vi "Data_1D_with_IgorX.vi"(6 "Data From Igor":bool, 8 "error in (no error)":errorcluster, 9 "Wave Name":string, 10 "Wave Prefix":string, 11 "1D Data IN":dbl[](array[numeric])) -> (0 "error out":errorcluster, 2 "Wave Prefix Through":string, 3 "1D Data OUT":dbl[](array[numeric]))   [LabVIEW 2014]
panel:
  in  "Igor Application IN":refnum<k7>
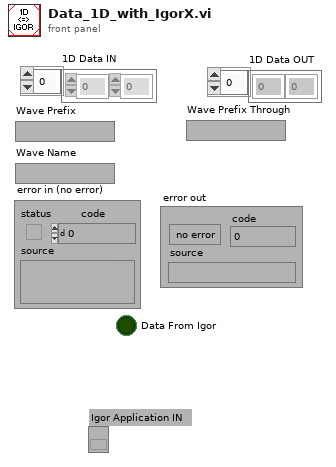
[diagram p1: front panel]
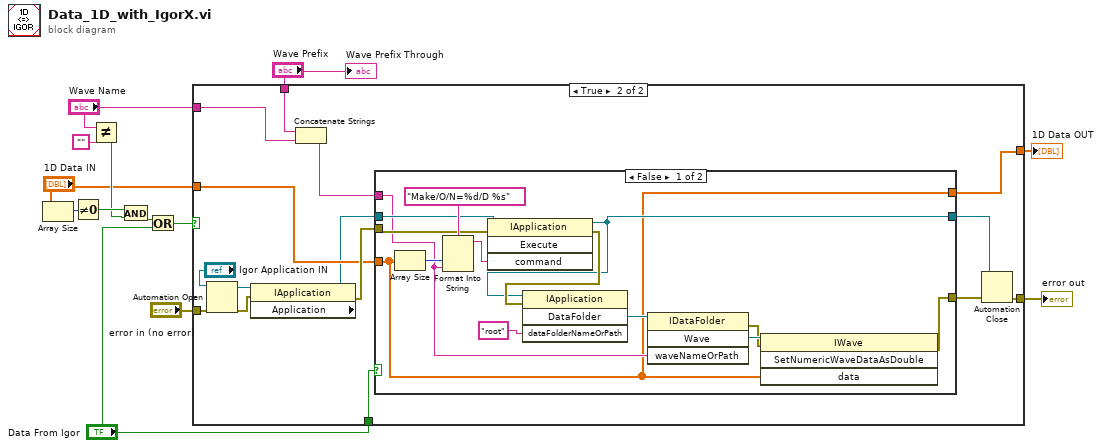
[diagram p0: block diagram]
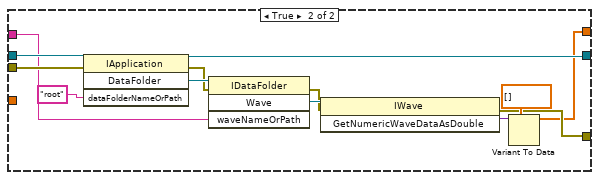
[diagram p3: hidden frame]
diagram:
  n1 = Array Size(array="1D Data IN") -> (size(s)=w13:i32)
  n2 = Not Equal To 0?(x=w13) -> (x != 0?=w12:bool)
  n3 = Not Equal?(x="Wave Name", y="") -> (x != y?=w9:bool)
  n4 = And(x=w12, y=w9) -> (x .and. y?=w3:bool)
  n5 = Or(x=w3, y="Data From Igor") -> (x .or. y?=w2:bool)
  n6 = case shown="True" w2 {
    tunnel: "1D Data IN" -> [w14 w17]
    tunnel: "Wave Name" -> [_ w29]
    tunnel: "Wave Prefix" -> [_ w30]
    tunnel: "error in (no error)" -> [w15 w24]
    tunnel: [w15 w22] -> w7
    tunnel: "Data From Igor" -> [_ w28]
    tunnel: [w14 w18] -> w4
    frame False {
    }
    frame True {
      n7 = Automation Open(error in (no error)=w24, Automation Refnum="Igor Application IN") -> (Automation Refnum=w25:refnum<k7>, error out=w27:errorcluster)  [unwired: 2 in]
      n8 = property class="IApplication"(reference=w25, error in=w27) -> (error out=w23:errorcluster, "Application"=w16:refnum<k7>)  [unwired: 1 out]
      n9 = Concatenate Strings(w30, w29) -> (w20:string)
      n10 = case shown="False" w28 {
        tunnel: w23 -> [w41 w50]
        tunnel: [w32 w46] -> w21
        tunnel: w16 -> [w42 w49]
        tunnel: w20 -> [w34 w48]
        tunnel: [w33 w47] -> w19
        tunnel: [w31 w45] -> w18
        tunnel: w17 -> [w31 _]
        frame False {
          n11 = Array Size(array=w31) -> (size(s)=w43:i32)
          n12 = Format Into String(format string="Make/O/N=%d/D %s" ("dataFolderNameOrPath"), w43, w34) -> (resulting string=w40:string)  [unwired: 2 in, 1 out]
          n13 = invoke class="IApplication" method="Execute"(reference=w42, error in=w41, "command"=w40) -> (reference out=w33:refnum<k7>, error out=w35:errorcluster)  [unwired: 1 in, 2 out]
          n14 = invoke class="IApplication" method="DataFolder"(reference=w33, error in=w35, "dataFolderNameOrPath"="root") -> ("DataFolder"=w36:refnum<k7>)  [unwired: 1 in, 3 out]
          n15 = invoke class="IDataFolder" method="Wave"(reference=w36, "waveNameOrPath"=w34) -> (error out=w37:errorcluster, "Wave"=w39:refnum<k7>)  [unwired: 2 in, 2 out]
          n16 = invoke class="IWave" method="SetNumericWaveDataAsDouble"(reference=w39, error in=w37, "data"=w31) -> (error out=w32:errorcluster)  [unwired: 1 in, 3 out]
        }
        frame True {
          n17 = invoke class="IApplication" method="DataFolder"(reference=w49, error in=w50, "dataFolderNameOrPath"="root") -> (reference out=w47:refnum<k7>, error out=w53:errorcluster, "DataFolder"=w54:refnum<k7>)  [unwired: 1 in, 1 out]
          n18 = invoke class="IDataFolder" method="Wave"(reference=w54, error in=w53, "waveNameOrPath"=w48) -> (error out=w55:errorcluster, "Wave"=w57:refnum<k7>)  [unwired: 1 in, 2 out]
          n19 = invoke class="IWave" method="GetNumericWaveDataAsDouble"(reference=w57, error in=w55) -> (error out=w46:errorcluster, "GetNumericWaveDataAsDouble"=w52:variant)  [unwired: 1 in, 1 out]
          n20 = Variant To Data(type=dbl[] [] ("1D Data IN"), Variant=w52) -> (data=w45:dbl[])  [unwired: 1 in, 1 out]
        }
      }
      n21 = Automation Close(3:w21, 5:w19) -> (0:w22:errorcluster)
    }
  }
  "error out" <- w7
  "1D Data OUT" <- w4
  "Wave Prefix Through" <- "Wave Prefix"
